vi "Start Task.vi"(8 "error in":errorcluster, 11 "NI PWM Input in":refnum<class "NI PWM Input.lvclass">) -> (0 "error out":errorcluster, 3 "NI PWM Input out":refnum<class "NI PWM Input.lvclass">)   [LabVIEW 2023, in "HardwareAbstractionLayer_LVOOP.lvlib" / "NI PWM Input.lvclass"]
doc: "This VI is DAQmx Start Task"
uses:
  NI PWM Input.lvclass
  NI PWM Input.lvclass/NI PWM Input.ctl
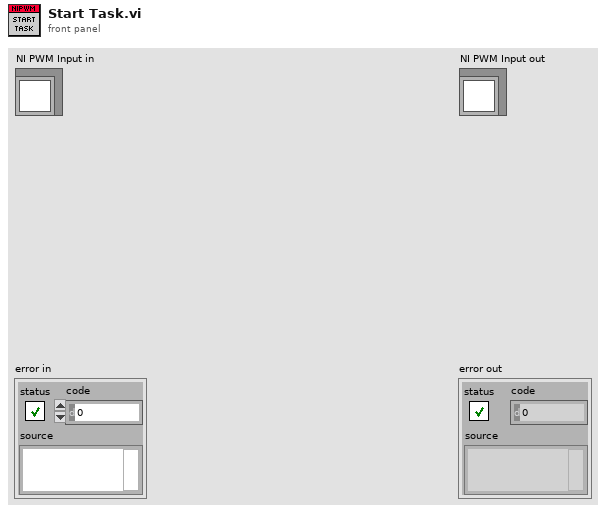
[diagram p1: front panel]
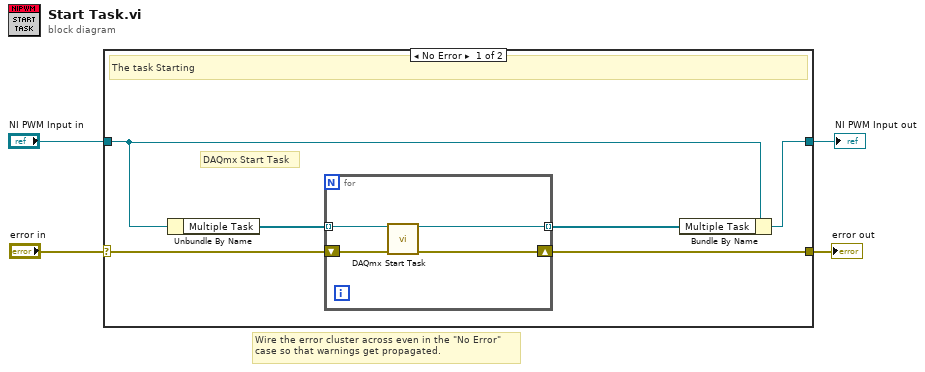
[diagram p0: block diagram]
diagram:
  # "Wire the error cluster across even in the \"No Error\"\ncase so that warnings get propagated."
  n1 = case shown="No Error" "error in" {
    selector: "error in" -> [w10 w16]
    tunnel: [w9 w16] -> w3
    tunnel: [w6 w15] -> w1
    tunnel: "NI PWM Input in" -> [w7 w15]
    frame No Error {
      # "DAQmx Start Task"
      # "The task Starting"
      n2 = Unbundle By Name(w7) -> ("Multiple Task"=w8:refnum<k21>[])
      n3 = for {
        tunnel: w8 -> [w12] mode=indexing
        tunnel: [w11] -> w5 mode=indexing
        shift-right: [w13] -> w9
        shift-left: w10 -> [w14]
        n4 = call <vilib>:"DAQmx Start Task.vi"("task/channels in"=w12, "error in"=w14) -> ("task out"=w11:refnum<k21>, "error out"=w13:errorcluster)  [unwired: 12 in]
      }
      n5 = Bundle By Name(cluster=w7, "Multiple Task"=w5) -> (w6:refnum<class "NI PWM Input.lvclass">)
    }
    frame Error {
    }
  }
  "error out" <- w3
  "NI PWM Input out" <- w1
